vi "IB_RW_Project_Source.vi"(7 "action":T3, 8 "error in (no error)":errorcluster, 9 "index in":string, 10 "dataSource in":T2, 11 "buildObject":T1) -> (0 "error out":errorcluster, 1 "index out":string, 2 "dataSource out":T2, 3 "buildObject out":T1)   [LabVIEW 2020]
doc: "Reads and writes the data to the object property bag."
uses:
  <resource>/Framework/Providers/API/ItemRef.ctl
  <vilib>/AppBuilder/IB_RW_Project/IB_RW_Project_Source_Data.ctl
  <vilib>/AppBuilder/IB_RW_Project/IB_RW_Project_PropBag_Action.ctl
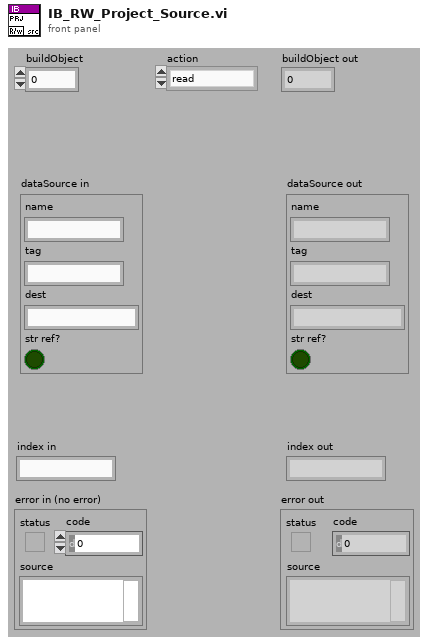
[diagram p1: front panel]
types:
  T1 = typedef "ItemRef.ctl" = u64
  T2 = typedef "IB_RW_Project_Source_Data.ctl" = cluster{"name":string, "tag":string, "dest":string, "str ref?":bool}
  T3 = typedef "IB_RW_Project_PropBag_Action.ctl" = enum16{"read", "write", "clear", "readPrevious", "writePrevious", "clearPrevious"}
  T4 = typedef "mxLvPropertyType.ctl" = enum32{"Unknown", "String", "Integer", "Binary", "Reference", "Double", "Unsigned Integer", "Boolean", "XML", "Path"}
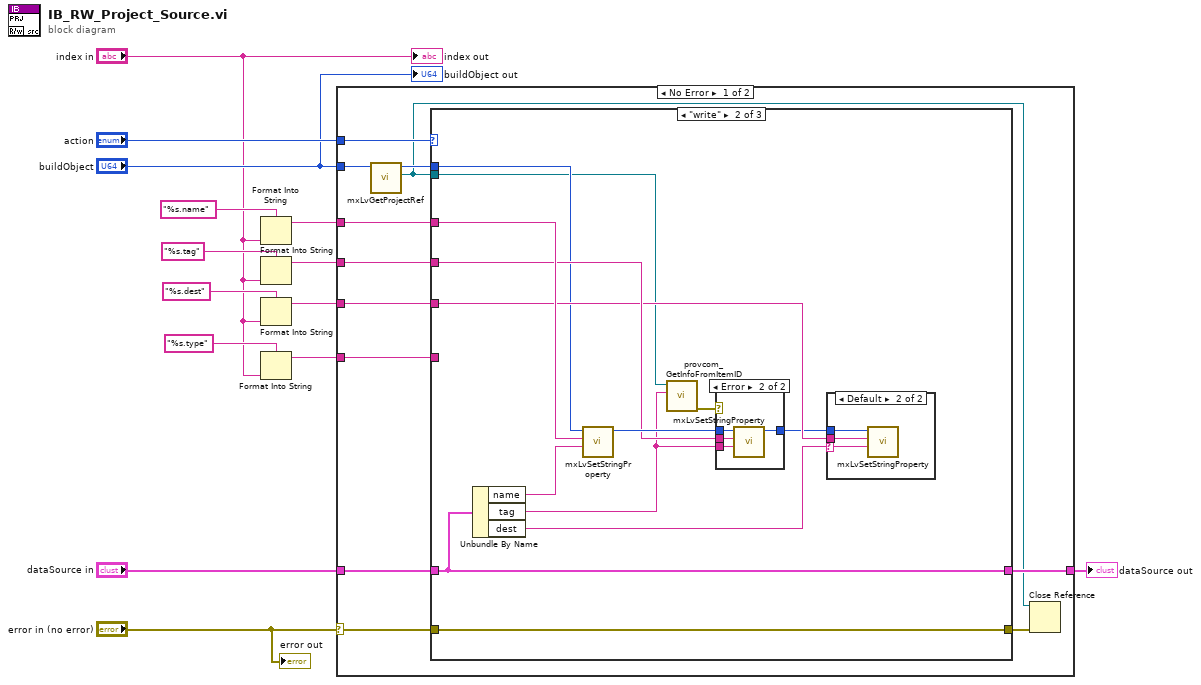
[diagram p0: block diagram]
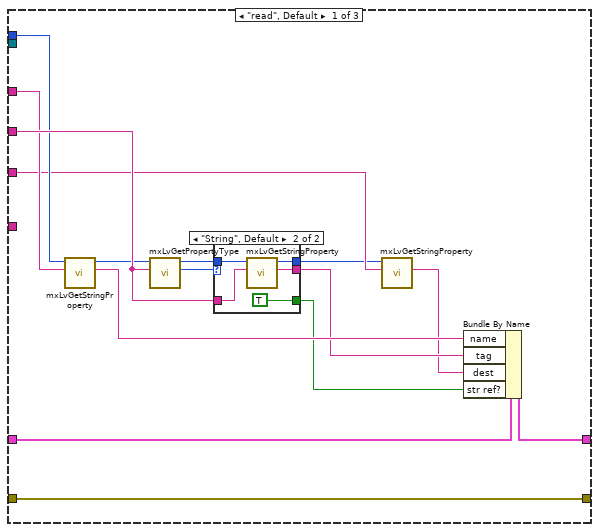
[diagram p2: hidden frame]
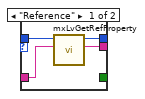
[diagram p3: hidden frame]
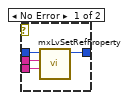
[diagram p5: hidden frame]
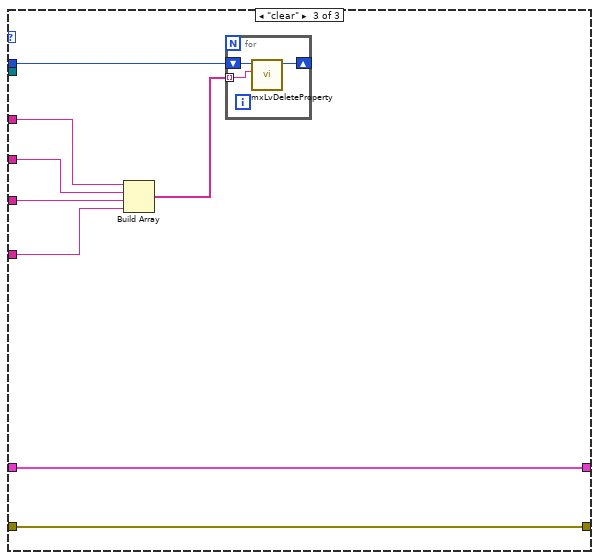
[diagram p6: hidden frame]
diagram:
  n1 = Format Into String(format string="%s.name", "index in") -> (resulting string=w8:string)  [unwired: 2 in, 1 out]
  n2 = Format Into String(format string="%s.tag", "index in") -> (resulting string=w6:string)  [unwired: 2 in, 1 out]
  n3 = Format Into String(format string="%s.dest", "index in") -> (resulting string=w4:string)  [unwired: 2 in, 1 out]
  n4 = Format Into String(format string="%s.type", "index in") -> (resulting string=w1:string)  [unwired: 2 in, 1 out]
  n5 = case shown="No Error" "error in (no error)" {
    selector: "error in (no error)" -> [w20 _]
    tunnel: "action" -> [w26 _]
    tunnel: "dataSource in" -> [w25 w86]
    tunnel: w8 -> [w24 _]
    tunnel: [w23 w86] -> w12
    tunnel: "buildObject" -> [w18 _]
    tunnel: w6 -> [w22 _]
    tunnel: w4 -> [w21 _]
    tunnel: w1 -> [w15 _]
    frame No Error {
      n6 = call <resource>:"mxLvGetProjectRef.vi"("Item"=w18) -> ("Project Refnum"=w16:refnum<vi>, "Item"=w17:T1)  [unwired: 1 in, 8 out]
      n7 = case shown="\"write\"" w26 {
        tunnel: w17 -> [w36 w53 w79]
        tunnel: w25 -> [w41 w63 w82]
        tunnel: w24 -> [w34 w60 w81]
        tunnel: [w40 w63 w82] -> w23
        tunnel: w22 -> [w37 w59 w80]
        tunnel: w21 -> [w31 w56 w77]
        tunnel: w20 -> [w28 w54 w76]
        tunnel: [w28 w54 w76] -> w19
        tunnel: w16 -> [_ w52 _]
        tunnel: w15 -> [_ _ w75]
        frame "read", Default {
          n8 = call <resource>:"mxLvGetStringProperty.vi"("Tag"=w34, "Item"=w36) -> ("Value"=w33:string, "Item"=w35:T1)  [unwired: 1 in, 7 out]
          n9 = call <resource>:"mxLvGetPropertyType.vi"("Tag"=w37, "Item"=w35) -> ("Type"=w39:T4, "Item"=w38:T1)  [unwired: 1 in, 7 out]
          n10 = case shown="\"String\", Default" w39 {
            tunnel: w38 -> [w45 w50]
            tunnel: w37 -> [w43 w49]
            tunnel: [w44 w48] -> w29
            tunnel: [w42 w47] -> w32
            tunnel: [_ TRUE] -> w27
            frame "Reference" {
              n11 = call <resource>:"mxLvGetRefProperty.vi"("Tag"=w43, "Item"=w45) -> ("Value"=w42:string, "Item"=w44:T1)  [unwired: 1 in, 7 out]
            }
            frame "String", Default {
              n12 = call <resource>:"mxLvGetStringProperty.vi"("Tag"=w49, "Item"=w50) -> ("Value"=w47:string, "Item"=w48:T1)  [unwired: 1 in, 7 out]
            }
          }
          n13 = call <resource>:"mxLvGetStringProperty.vi"("Tag"=w31, "Item"=w29) -> ("Value"=w30:string)  [unwired: 1 in, 8 out]
          n14 = Bundle By Name(cluster=w41, "name"=w33, "tag"=w32, "dest"=w30, "str ref?"=w27) -> (w40:T2)
        }
        frame "write" {
          n15 = Unbundle By Name(w63) -> ("name"=w58:string, "tag"=w57:string, "dest"=w51:string)
          n16 = call <resource>:"mxLvSetStringProperty.vi"("Value (\"\")"=w58, "Tag"=w60, "Item"=w53) -> ("Item"=w61:T1)  [unwired: 2 in, 6 out]
          n17 = call <resource>:"provcom_GetInfoFromItemID.vi"("ItemID"=w57, "Project"=w52) -> ("ErrOut"=w62:errorcluster)  [unwired: 1 in, 8 out]
          n18 = case shown="Error" w62 {
            tunnel: w61 -> [w70 w74]
            tunnel: [w69 w73] -> w55
            tunnel: w59 -> [w68 w72]
            tunnel: w57 -> [w67 w71]
            frame No Error {
              n19 = call <resource>:"mxLvSetRefProperty.vi"("Value (\"\")"=w67, "Tag"=w68, "Item"=w70) -> ("Item"=w69:T1)  [unwired: 2 in, 6 out]
            }
            frame Error {
              n20 = call <resource>:"mxLvSetStringProperty.vi"("Value (\"\")"=w71, "Tag"=w72, "Item"=w74) -> ("Item"=w73:T1)  [unwired: 2 in, 6 out]
            }
          }
          n21 = case shown="Default" w51 {
            selector: w51 -> [_ w64]
            tunnel: w56 -> [_ w66]
            tunnel: w55 -> [_ w65]
            frame "" {
            }
            frame Default {
              n22 = call <resource>:"mxLvSetStringProperty.vi"("Value (\"\")"=w64, "Tag"=w66, "Item"=w65) -> ()  [unwired: 2 in, 7 out]
            }
          }
        }
        frame "clear" {
          n23 = Build Array(w81, w80, w77, w75) -> (w78:string[])
          n24 = for {
            shift-right: [w85] -> _
            shift-left: w79 -> [w84]
            tunnel: w78 -> [w83] mode=indexing
            n25 = call <resource>:"mxLvDeleteProperty.vi"("Tag"=w83, "Item"=w84) -> ("Item"=w85:T1)  [unwired: 1 in, 8 out]
          }
        }
      }
      n26 = Close Reference(reference=w16, error in (no error)=w19) -> ()  [unwired: 1 out]
    }
    frame Error {
    }
  }
  "dataSource out" <- w12
  "error out" <- "error in (no error)"
  "buildObject out" <- "buildObject"
  "index out" <- "index in"
